vi "CopyFile.vi"(8 "error in (no error)":errorcluster, 10 "System Status Ref.":refnum<vi>, 11 "Source File":path[](array[path])) -> (0 "error out":errorcluster, 3 "Source File dup.":path)   [LabVIEW 2015, in "CopyUtility.lvlib"]
uses:
  CopyUtility.lvlib
  ConfigHelper/ConfigHelper.lvlib
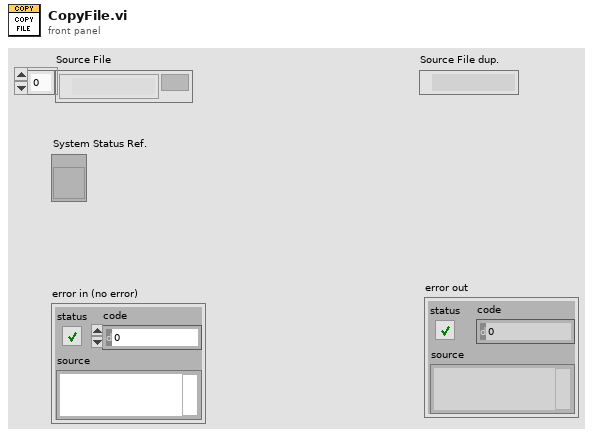
[diagram p1: front panel]
types:
  T1 = typedef "ConfigHelper.lvlib/Config.ctl" = cluster{"Path":string, "Days to Keep":i32, "Number of Rows":i32}
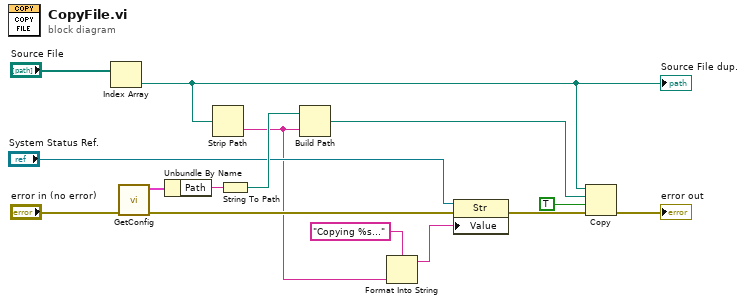
[diagram p0: block diagram]
diagram:
  n1 = Index Array(array="Source File") -> (element=w12:path)  [unwired: 1 in]
  "Source File dup." <- w12
  n2 = call "GetConfig.vi"("error in (no error)"="error in (no error)") -> ("error out"=w6:errorcluster, "Config"=w10:T1)  [unwired: 9 in]
  n3 = Unbundle By Name(w10) -> ("Path"=w9:string)
  n4 = Strip Path(path=w12) -> (name=w2:string)  [unwired: 1 out]
  n5 = String To Path(string=w9) -> (path=w8:path)
  n6 = Build Path(base path=w8, name or relative path=w2) -> (appended path=w14:path)
  n7 = Format Into String(format string="Copying %s...", w2) -> (resulting string=w1:string)  [unwired: 2 in, 1 out]
  n8 = property class="Str"(reference="System Status Ref.", error in=w6, "Value"=w1) -> (error out=w5:errorcluster)  [unwired: 1 out]
  n9 = Copy(8:w5, 9:TRUE ("overwrite (F)"), 10:w14, 11:w12) -> (0:→"error out":errorcluster)  [unwired: 1 in, 2 out]
